vi "locate enable tag.vi"(10 "bin datalogger configuration":refnum<class "Binary datalogger configuration.lvclass">, 11 "data dictionary in":refnum<class "data dictionary.lvclass">) -> (1 "found?":bool, 2 "index":i32, 3 "data dictionary out":refnum<class "data dictionary.lvclass">)   [LabVIEW 2013, in "Binary datalogger runtime.lvclass"]
uses:
  Binary datalogger runtime.lvclass
  <vilib>/NI/Tag Bus/dictionary/data dictionary.lvclass
  configuration/Binary datalogger configuration.lvclass
  <vilib>/NI/Tag Bus/tag/tag descriptor.lvclass/tag descriptor.ctl
  <vilib>/NI/Tag Bus/tag/read tag name.vi
  <vilib>/NI/Tag Bus/tag/read data type.vi
  <vilib>/NI/Tag Bus/dictionary/locate tag.vi
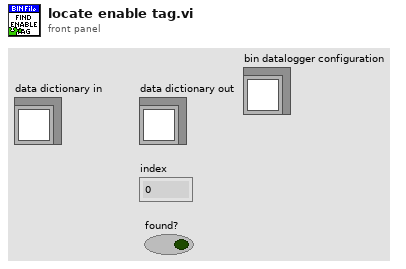
[diagram p1: front panel]
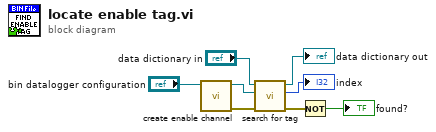
[diagram p0: block diagram]
diagram:
  n1 = call "create enable channel.vi"("bin datalogger configuration"="bin datalogger configuration") -> ("error out"=w3:errorcluster, "enable channel"=w2:refnum<class "TBM channel.lvclass">)  [unwired: 8 in, 1 out]
  n2 = call <vilib>:"search for tag.vi"("error in"=w3, "system tag"=w2, "data dictionary in"="data dictionary in") -> ("error out"=w7:errorcluster, "index"=→"index":i32, "data dictionary out"=→"data dictionary out":refnum<class "data dictionary.lvclass">)  [unwired: 6 in]
  n3 = Not(x=w7) -> (.not. x?=→"found?":bool)
